vi "Close.vi"(8 "error in (no error)":errorcluster, 11 "Camera Base in":refnum<class "Camera Base.lvclass">) -> (0 "error out":errorcluster, 3 "Camera Base out":refnum<class "Camera Base.lvclass">)   [LabVIEW 2023, in "Camera Base.lvclass"]
uses:
  Camera Base.lvclass
  Camera Base.lvclass/Camera Base.ctl
  Interfaces/IConfigure/IConfigure.lvclass
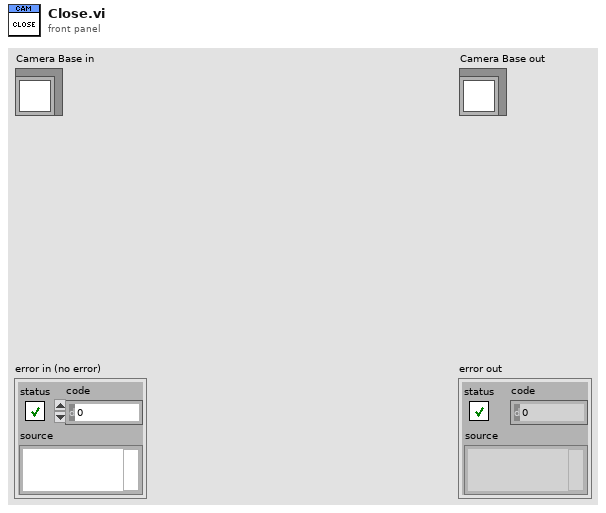
[diagram p1: front panel]
types:
  T1 = typedef "IMAQ Image.ctl" = refnum<image>
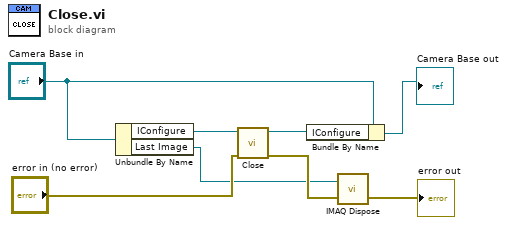
[diagram p0: block diagram]
diagram:
  n1 = Unbundle By Name("Camera Base in") -> ("IConfigure"=w7:refnum<class "IConfigure.lvclass">, "Last Image"=w2:T1)
  n2 = call-dynamic "Close.vi"("error in"="error in (no error)", "IConfigure in"=w7) -> ("error out"=w3:errorcluster, "IConfigure out"=w4:refnum<class "IConfigure.lvclass">)  [unwired: 8 in]
  n3 = Bundle By Name(cluster="Camera Base in", "IConfigure"=w4) -> (→"Camera Base out":refnum<class "Camera Base.lvclass">)
  n4 = call "IMAQ Dispose"("Image"=w2, "error in (no error)"=w3) -> ("error out"=→"error out":errorcluster)  [unwired: 4 in]
